vi "PCO_GetImageTiming.vi"(8 "error in (no error)":errorcluster {"code" format="%x"}, 11 "ph":u64) -> (0 "error out":errorcluster {"code" format="%x"}, 1 "strImageTiming":T1, 2 "ErrorMessage":i32 format="%x", 3 "ph out":u64)   [LabVIEW 2019, in "SDK.lvlib" / "TimingControl.lvlib"]
doc: "<b>Description:</b>\nThis function returns the current image timing in nanosecond resolution and additional trigger system information.\nThe command will be rejected, if Recording State is [run], see PCO_GetRecordingState.\n\nThe maximum real trigger delay in ns can be calculated as: \nReal Trigger Delay = TriggerSystemDelay_ns + TriggerSystemJitter_ns + \n TriggerDelay_ns + TriggerDelay_s*1000000000\n\nThe minimum real trigger delay in ns can be calculated as: \nReal Trigger Delay = TriggerSystemDelay_ns + 0 + \n TriggerDelay_ns + TriggerDelay_s*1000000000\n\n<b>Supported camera type:</b>\npco.edge\n\n<b>Descriptor dependency:</b>\nNone"
uses:
  TimingControl.lvlib
  Structures/Structures.lvlib
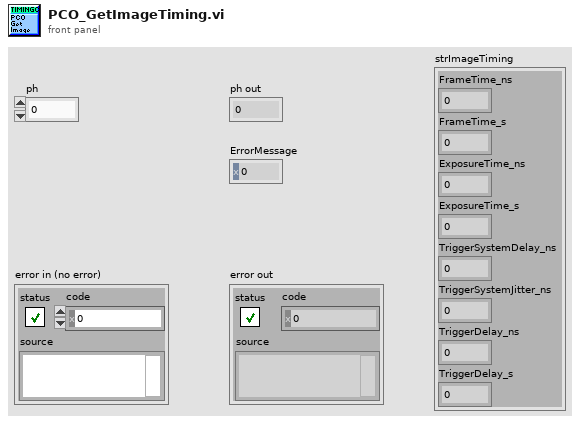
[diagram p1: front panel]
types:
  T1 = cluster{"FrameTime_ns":u32, "FrameTime_s":u32, "ExposureTime_ns":u32, "ExposureTime_s":u32, "TriggerSystemDelay_ns":u32, "TriggerSystemJitter_ns":u32, "TriggerDelay_ns":u32, "TriggerDelay_s":u32}
  T2 = cluster{"wSize":u16, "wDummy":u16, "FrameTime_ns":u32, "FrameTime_s":u32, "ExposureTime_ns":u32, "ExposureTime_s":u32, "TriggerSystemDelay_ns":u32, "TriggerSystemJitter_ns":u32, "TriggerDelay_ns":u32, "TriggerDelay_s":u32, "ZZdwDummy":cluster{u32, u32, u32, u32, u32, u32, u32, u32, u32, u32, u32}}
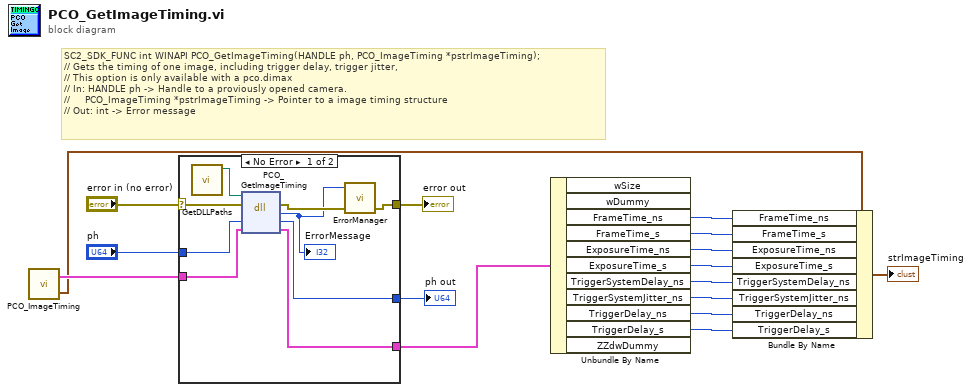
[diagram p0: block diagram]
diagram:
  # "SC2_SDK_FUNC int WINAPI PCO_GetImageTiming(HANDLE ph, PCO_ImageTiming *pstrImageTiming);\n// Gets the timing of one image, including trigger delay, trigger jitter, \n// This option is only available with a pco.dimax\n// In: HANDLE ph -> Handle to a proviously opened camera.\n//     PCO_ImageTiming *pstrImageTiming -> Pointer to a image timing structure\n// Out: int -> Error message"
  n1 = call "PCO_ImageTiming.vi"() -> ("PCO_ImageTiming"=w10:T1, "PCO_ImageTiming_Raw"=w12:T2)  [unwired: 4 in, 2 out]
  n2 = case shown="No Error" "error in (no error)" {
    selector: "error in (no error)" -> [w21 w28]
    tunnel: "ph" -> [w25 w27]
    tunnel: [w24 w27] -> w15
    tunnel: w12 -> [w23 w26]
    tunnel: [w22 w26] -> w11
    tunnel: [w19 w28] -> w14
    frame No Error {
      n3 = call "GetDLLPaths.vi"() -> ("SC2_Cam_Path"=w17:path)  [unwired: 8 in, 3 out]
      n4 = dll-call lib="?" fn="PCO_GetImageTiming"(path in=w17, error in=w21, "ph"=w25, "pstrImageTiming"=w23) -> (error out=w20:errorcluster, "return type"=w18:i32, "ph"=w24:u64, "pstrImageTiming"=w22:T2)  [unwired: 1 in, 1 out]
      "ErrorMessage" <- w18
      n5 = call "ErrorManager.vi"("error in (no error)"=w20, "error code"=w18) -> ("error out"=w19:errorcluster)  [unwired: 2 in, 1 out]
    }
    frame Error {
    }
  }
  "ph out" <- w15
  "error out" <- w14
  n6 = Unbundle By Name(w11) -> ("FrameTime_ns"=w9:u32, "FrameTime_s"=w8:u32, "ExposureTime_ns"=w7:u32, "ExposureTime_s"=w6:u32, "TriggerSystemDelay_ns"=w5:u32, "TriggerSystemJitter_ns"=w4:u32, "TriggerDelay_ns"=w3:u32, "TriggerDelay_s"=w2:u32)  [unwired: 3 out]
  n7 = Bundle By Name(cluster=w10, "FrameTime_ns"=w9, "FrameTime_s"=w8, "ExposureTime_ns"=w7, "ExposureTime_s"=w6, "TriggerSystemDelay_ns"=w5, "TriggerSystemJitter_ns"=w4, "TriggerDelay_ns"=w3, "TriggerDelay_s"=w2) -> (→"strImageTiming":T1)
